vi "CV_read_open_correction.vi"(8 "error in":errorcluster, 11 "Input parameters in":T1={"Measurement type"=enum."Debug", "Sensor type"=enum."HPK_8in_256", "Identifier"="test.txt", "Open after execution?"=FALSE, "Plot after execution?"=FALSE, "Display channel"=0, "Voltage Delay (s)"=0.5, "Switch Delay (s)"=0.01, "VISA resource name source"="", "VISA resource name DMM"="", "VISA resource name LCR"="", "Compliance  Level (A)"=10.0, "Voltage Limit (V)"=1000.0, "Data storage location"="", "Scan voltages"="", "Use source as DMM?"=FALSE, "LCR signal frequenzy (Hz)"=10.0, "DMM device"=enum."Keithley2001", "Sampling number"=1, "Use env. sensors on"=enum."Sensirion sht1x/7x", "Switchboard Handle"=0, "Use Switchboard"=FALSE, "LCR signal voltage (V)"=10000.0, "Repeat"=1, "Scan voltages IV"="", "Scan voltages CV"="", "Hex pad numbers?"=FALSE, "Set measurement type"=enum."Debug", "Custom pad scan"="", "IV voltage Delay (s)"=0.5, "CV voltage Delay (s)"=0.5, "Needle measurement?"=FALSE, "Comments"="test.txt", "LCR signal frequenzy (kHz)"=10.0, "Compliance  Level (uA)"=10.0, "Open Correction Array"=array2304x3[6912 elements], "Current set voltage"=0.0, "Last set voltage"=0.0, "Current channel"=0, "Last OpenCorrection index"=-1, "Total curr/vltg every x steps"=10, "Current channel iteration"=0, "No CV corrections"=FALSE, "Mapfile"="", "Corrfile"="", "IV voltage file"=path "", "CV voltage file"=path "", "IV Switch Delay (s)"=0.01, "CV Switch Delay (s)"=0.01} {"CV Switch Delay (s)" format="%#_13g"; "IV Switch Delay (s)" format="%#_13g"; "Last set voltage" format="%#_13g"; "Current set voltage" format="%#_13g"; "CV voltage Delay (s)" format="%#_13g"; "IV voltage Delay (s)" format="%#_13g"; "Voltage Limit (V)" format="%#_13g"; "Voltage Delay (s)" format="%#_13g"; "Switch Delay (s)" format="%#_13g"}) -> (0 "error out":errorcluster, 3 "Input parameters out":T1={"Measurement type"=enum."Debug", "Sensor type"=enum."HPK_8in_256", "Identifier"="test.txt", "Open after execution?"=FALSE, "Plot after execution?"=FALSE, "Display channel"=0, "Voltage Delay (s)"=0.5, "Switch Delay (s)"=0.01, "VISA resource name source"="", "VISA resource name DMM"="", "VISA resource name LCR"="", "Compliance  Level (A)"=10.0, "Voltage Limit (V)"=1000.0, "Data storage location"="", "Scan voltages"="", "Use source as DMM?"=FALSE, "LCR signal frequenzy (Hz)"=10.0, "DMM device"=enum."Keithley2001", "Sampling number"=1, "Use env. sensors on"=enum."Sensirion sht1x/7x", "Switchboard Handle"=0, "Use Switchboard"=FALSE, "LCR signal voltage (V)"=10000.0, "Repeat"=1, "Scan voltages IV"="", "Scan voltages CV"="", "Hex pad numbers?"=FALSE, "Set measurement type"=enum."Debug", "Custom pad scan"="", "IV voltage Delay (s)"=0.5, "CV voltage Delay (s)"=0.5, "Needle measurement?"=FALSE, "Comments"="test.txt", "LCR signal frequenzy (kHz)"=10.0, "Compliance  Level (uA)"=10.0, "Open Correction Array"=array2304x3[6912 elements], "Current set voltage"=0.0, "Last set voltage"=0.0, "Current channel"=0, "Last OpenCorrection index"=-1, "Total curr/vltg every x steps"=10, "Current channel iteration"=0, "No CV corrections"=FALSE, "Mapfile"="", "Corrfile"="", "IV voltage file"=path "", "CV voltage file"=path "", "IV Switch Delay (s)"=0.01, "CV Switch Delay (s)"=0.01} {"CV Switch Delay (s)" format="%#_13g"; "IV Switch Delay (s)" format="%#_13g"; "Last set voltage" format="%#_13g"; "Current set voltage" format="%#_13g"; "CV voltage Delay (s)" format="%#_13g"; "IV voltage Delay (s)" format="%#_13g"; "Voltage Limit (V)" format="%#_13g"; "Voltage Delay (s)" format="%#_13g"; "Switch Delay (s)" format="%#_13g"})   [LabVIEW 2016]
uses:
  input_params.ctl
panel:
  out "output array":dbl[][](array[numeric])
  out "array":string[][](array[string])
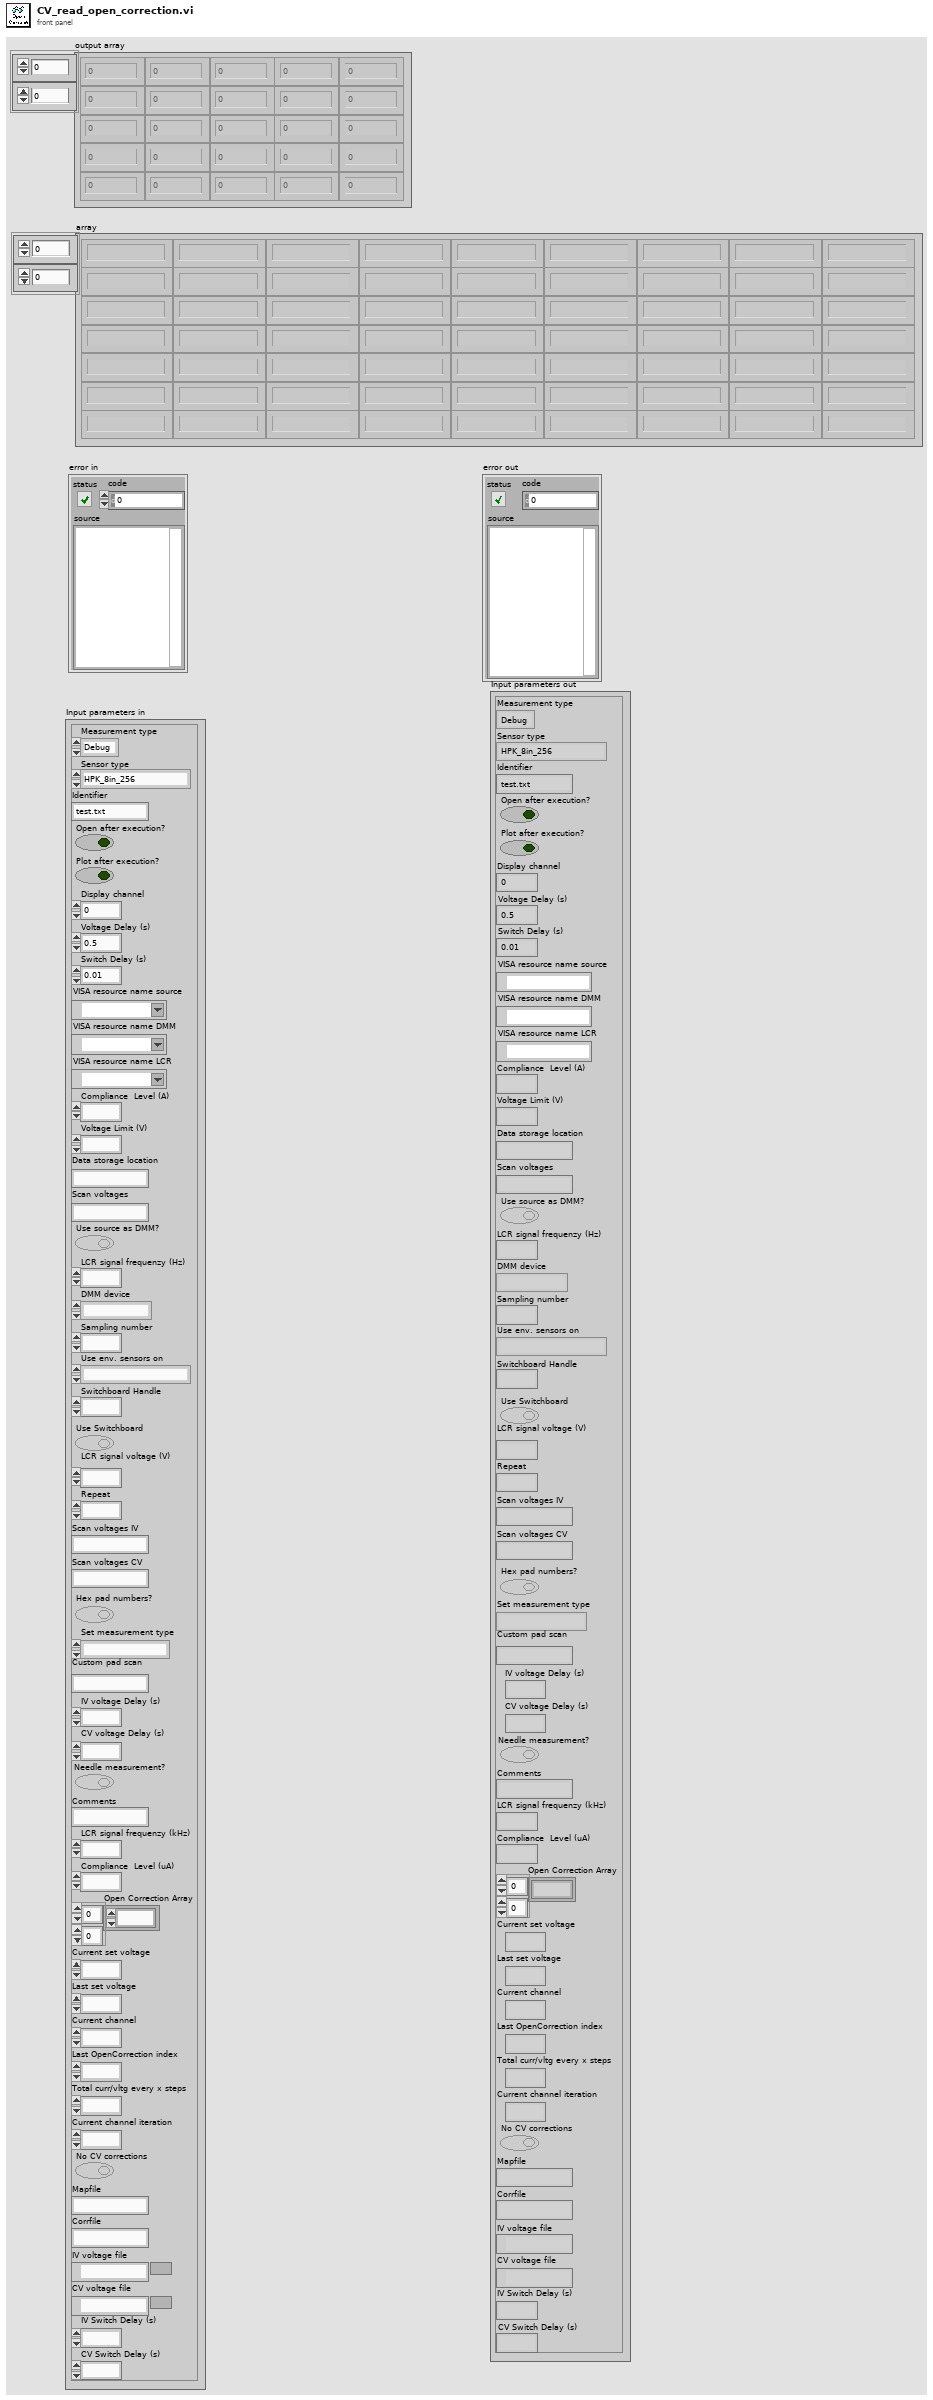
[diagram p1: front panel]
types:
  T1 = typedef "input_params.ctl" = cluster{"Measurement type":enum16{"IV", "CV", "Debug", "Test_contact"}, "Sensor type":enum16{"HPK_6in_135", "HPK_8in_256", "IFX_8in_256", "Diode", "HPK_6in_256", "Full matrix"}, "Identifier":string, "Open after execution?":bool, "Plot after execution?":bool, "Display channel":i32, "Voltage Delay (s)":dbl, "Switch Delay (s)":dbl, "VISA resource name source":refnum<visa-resource-name>, "VISA resource name DMM":refnum<visa-resource-name>, "VISA resource name LCR":refnum<visa-resource-name>, "Compliance  Level (A)":dbl, "Voltage Limit (V)":dbl, "Data storage location":string, "Scan voltages":string, "Use source as DMM?":bool, "LCR signal frequenzy (Hz)":dbl, "DMM device":enum16{"Keithley2001", "Keithley2450", "Keithley2410", "Keithley6487"}, "Sampling number":i32, "Use env. sensors on":enum16{"Sensirion sht1x/7x", "Switch Matrix", "Probecard"}, "Switchboard Handle":u32, "Use Switchboard":bool, "LCR signal voltage (V)":dbl, "Repeat":i32, "Scan voltages IV":string, "Scan voltages CV":string, "Hex pad numbers?":bool, "Set measurement type":enum16{"IV", "CV", "Debug", "Test_contact", "IV+CV"}, "Custom pad scan":string, "IV voltage Delay (s)":dbl, "CV voltage Delay (s)":dbl, "Needle measurement?":bool, "Comments":string, "LCR signal frequenzy (kHz)":dbl, "Compliance  Level (uA)":dbl, "Open Correction Array":dbl[][], "Current set voltage":dbl, "Last set voltage":dbl, "Current channel":i32, "Last OpenCorrection index":i32, "Total curr/vltg every x steps":i32, "Current channel iteration":i32, "No CV corrections":bool, "Mapfile":string, "Corrfile":string, "IV voltage file":path, "CV voltage file":path, "IV Switch Delay (s)":dbl, "CV Switch Delay (s)":dbl}
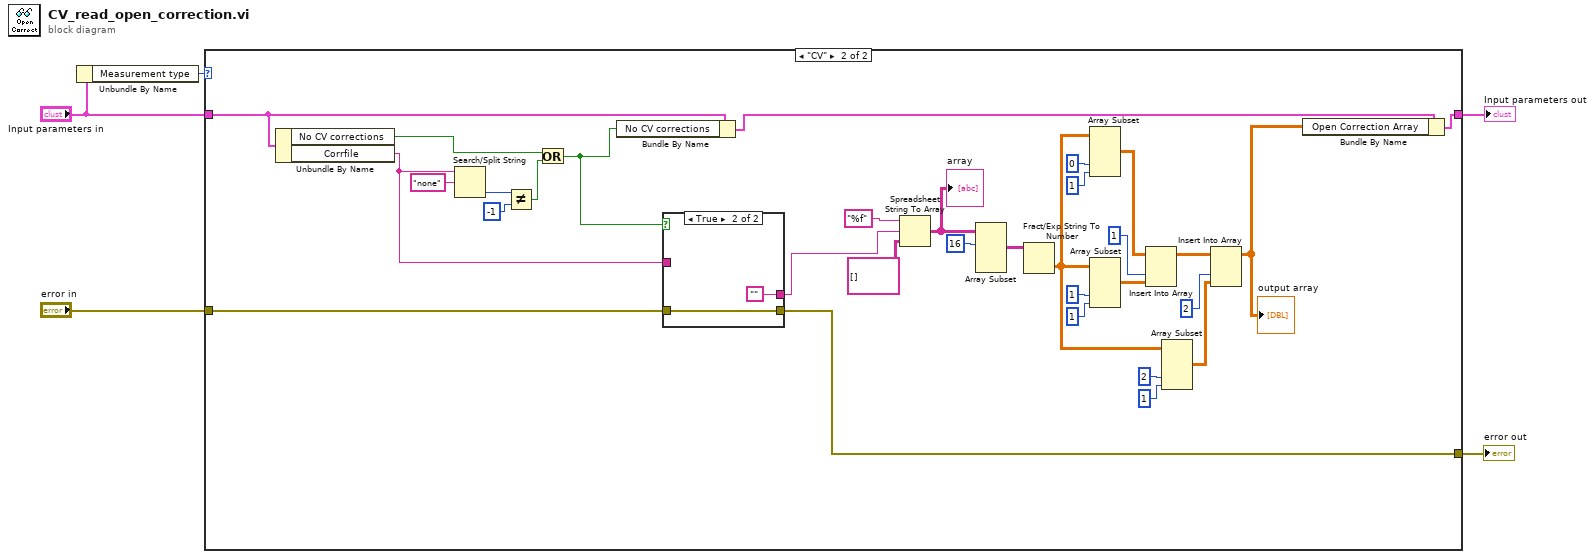
[diagram p0: block diagram]
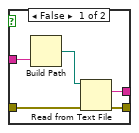
[diagram p3: hidden frame]
diagram:
  n1 = Unbundle By Name("Input parameters in") -> ("Measurement type"=w1:enum16{"IV", "CV", "Debug", "Test_contact"})
  n2 = case shown="\"CV\"" w1 {
    tunnel: "error in" -> [w6 w20]
    tunnel: [w6 w19] -> w4
    tunnel: [w7 w18] -> w3
    tunnel: "Input parameters in" -> [w7 w8]
    frame "IV", Default {
    }
    frame "CV" {
      n3 = Unbundle By Name(w8) -> ("No CV corrections"=w11:bool, "Corrfile"=w16:string)
      n4 = Search/Split String(string=w16, search string/char (-)="none") -> (offset of match=w14:i32)  [unwired: 1 in, 2 out]
      n5 = Not Equal?(x=w14, y=-1) -> (x != y?=w10:bool)
      n6 = Or(x=w11, y=w10) -> (x .or. y?=w9:bool)
      n7 = Bundle By Name(cluster=w8, "No CV corrections"=w9) -> (w12:T1)
      n8 = case shown="True" w9 {
        tunnel: [w43 ""] -> w39
        tunnel: w20 -> [w42 w46]
        tunnel: [w41 w46] -> w19
        tunnel: w16 -> [w40 _]
        frame False {
          n9 = Build Path(name or relative path=w40) -> (appended path=w44:path)  [unwired: 1 in]
          n10 = Read from Text File(file (use dialog)=w44, error in=w42) -> (text=w43:string, error out=w41:errorcluster)  [unwired: 2 in, 2 out]
        }
        frame True {
        }
      }
      n11 = Spreadsheet String To Array(format string="%f", spreadsheet string=w39, array type (2D Dbl)=string[][] [] ("Array")) -> (array=w35:string[][])  [unwired: 1 in]
      "array" <- w35
      n12 = Array Subset(array=w35, index (row)=16 ("index")) -> (w34:string[][])  [unwired: 3 in]
      n13 = Fract/Exp String To Number(string=w34) -> (number=w22:dbl[][])  [unwired: 3 in, 1 out]
      n14 = Array Subset(array=w22, index (col)=0 ("index"), length (col)=1 ("length")) -> (w31:dbl[][])  [unwired: 2 in]
      n15 = Array Subset(array=w22, index (col)=1 ("index"), length (col)=1 ("length")) -> (w28:dbl[][])  [unwired: 2 in]
      n16 = Insert Into Array(array=w31, index (col)=1 ("index (row)"), new element=w28) -> (w25:dbl[][])  [unwired: 1 in]
      n17 = Array Subset(array=w22, index (col)=2 ("index"), length (col)=1 ("length")) -> (w21:dbl[][])  [unwired: 2 in]
      n18 = Insert Into Array(array=w25, index (col)=2 ("index (row)"), new element=w21) -> (w17:dbl[][])  [unwired: 1 in]
      "output array" <- w17
      n19 = Bundle By Name(cluster=w12, "Open Correction Array"=w17) -> (w18:T1)
    }
  }
  "error out" <- w4
  "Input parameters out" <- w3
